vi "Board Add Player.vi"(8 "error in (no error)":errorcluster, 10 "Player":refnum<class "Player.lvclass">, 11 "Board in":refnum<class "Board.lvclass">) -> (0 "error out":errorcluster, 3 "Board out":refnum<class "Board.lvclass">)   [LabVIEW 2019, in "Board.lvclass"]
uses:
  Board.lvclass
  Player/Player.lvclass
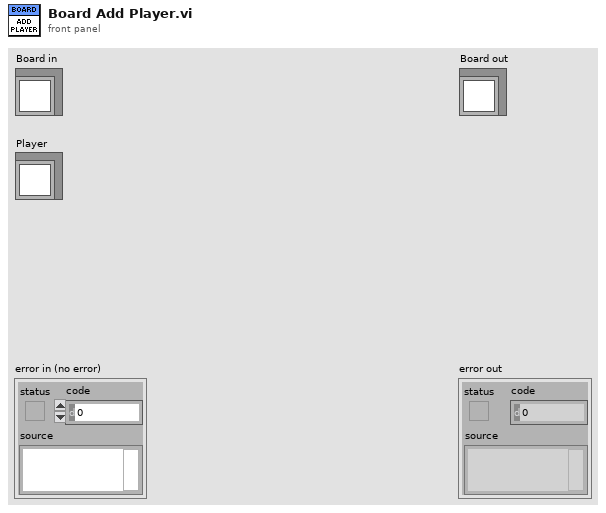
[diagram p1: front panel]
types:
  T1 = typedef "Coordinate STYP.ctl" = cluster{"X":i32, "Y":i32}
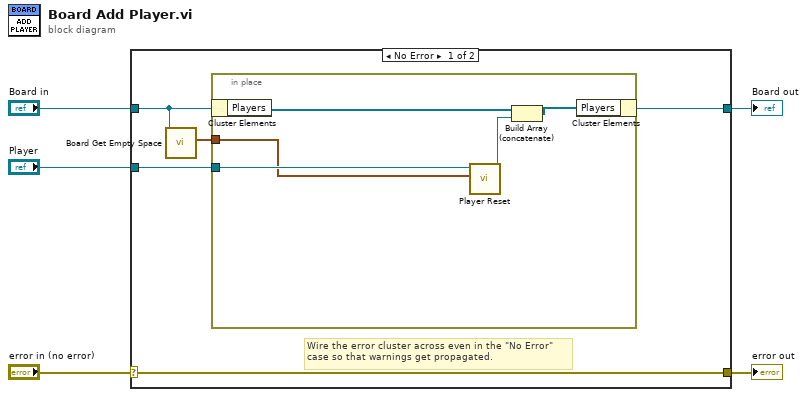
[diagram p0: block diagram]
diagram:
  n1 = case shown="No Error" "error in (no error)" {
    selector: "error in (no error)" -> [w10 w17]
    tunnel: [w10 w17] -> w4
    tunnel: [w9 w16] -> w2
    tunnel: "Board in" -> [w7 w16]
    tunnel: "Player" -> [w8 _]
    frame No Error {
      # "Wire the error cluster across even in the \"No Error\"\ncase so that warnings get propagated."
      n2 = call-dynamic "Board Get Empty Space.vi"("Board in"=w7) -> ("Coordinate"=w6:T1)  [unwired: 8 in, 2 out]
      n3 = in-place {
        in-place-border: w8 -> [w12]
        in-place-border: w6 -> [w11]
        n4 = in-place-cluster #1(w7) -> ("Players"=w15:refnum<class "Player.lvclass">[])
        n5 = call-dynamic "Player Reset.vi"("Starting Coordinate"=w11, "Player in"=w12) -> ("Player out"=w13:refnum<class "Player.lvclass">)  [unwired: 8 in, 1 out]
        n6 = Build Array (concatenate)(w15, w13) -> (w14:refnum<class "Player.lvclass">[])
        n7 = in-place-cluster #1("Players"=w14) -> (w9:refnum<class "Board.lvclass">)
      }
    }
    frame Error {
    }
  }
  "error out" <- w4
  "Board out" <- w2
